vi "Unitary matrix.vi"(9 "Final state? (T)":bool=TRUE, 11 "Circuit cluster":T2) -> (3 "Unitary matrix":T1)   [LabVIEW 2016]
uses:
  TypeDefs/Circuit Cluster.ctl
  Classes/GateAbst/GateAbst.lvclass
  <vilib>/Analysis/Matrix/Datatypes/ComplexMatrix.ctl
  <vilib>/Analysis/Matrix/NI_Matrix.lvlib
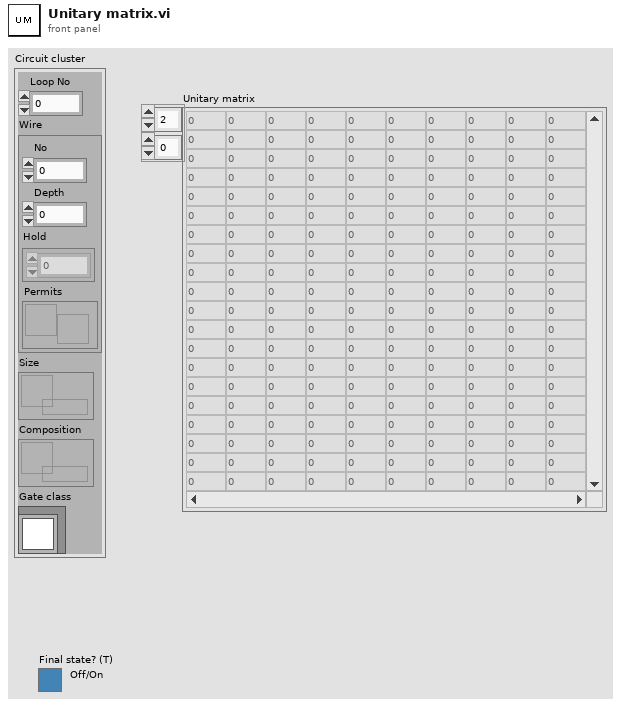
[diagram p1: front panel]
types:
  T1 = typedef "NI_Matrix.lvlib/ComplexMatrix.ctl" = cdb[][]
  T2 = typedef "Circuit Cluster.ctl" = cluster{"Loop No":i32, "Wire":cluster{"No":i32, "Depth":i32, "Hold":i32[][], "Permits":refnum<notifier>}, "Size":refnum<queue>, "Composition":refnum<queue>, "Gate class":refnum<class "GateAbst.lvclass">}
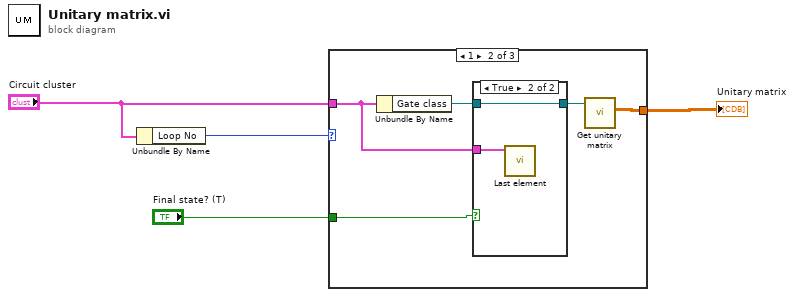
[diagram p0: block diagram]
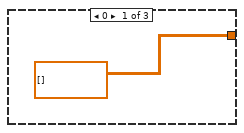
[diagram p2: hidden frame]
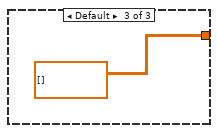
[diagram p4: hidden frame]
diagram:
  n1 = Unbundle By Name("Circuit cluster") -> ("Loop No"=w1:i32)
  n2 = case shown="1" w1 {
    tunnel: "Circuit cluster" -> [_ w7 _]
    tunnel: [T1 [] ("Unitary matrix") w10 T1 [] ("Unitary matrix")] -> w3
    tunnel: "Final state? (T)" -> [_ w6 _]
    frame 0 {
    }
    frame 1 {
      n3 = Unbundle By Name(w7) -> ("Gate class"=w9:refnum<class "GateAbst.lvclass">)
      n4 = case shown="True" w6 {
        tunnel: w9 -> [w11 w13]
        tunnel: [w11 w13] -> w8
        tunnel: w7 -> [_ w12]
        frame False {
        }
        frame True {
          n5 = call "Last element.vi"("Circuit cluster"=w12) -> ()  [unwired: 10 in, 1 out]
        }
      }
      n6 = call-dynamic "Get unitary matrix.vi"("GateAbst in"=w8) -> ("Unitary matrix"=w10:T1)  [unwired: 8 in, 2 out]
    }
    frame Default {
    }
  }
  "Unitary matrix" <- w3
